vi "EXA SweepLoop.vi"(0 "Session In":refnum<visa-resource-name>="TCPIP0::169.254.70.120::inst0::INSTR", 1 "AVG":i32=4, 5 "Fstart":dbl=20.0 caption="RF_FREQ", 7 "Fstop":dbl=40.0 caption="RF_FREQ", 9 "Span(MHz)":dbl=1000.0, 11 "error in":errorcluster {"code" format="%.0x"}, 12 "RBW(Hz)":string="30") -> (3 "Max Freq/Ampl":dbl[](array[numeric]), 4 "VISA resource name out":refnum<visa-resource-name>, 15 "error out":errorcluster)   [LabVIEW 2018]
uses:
  Agilent MXA Series/Agilent MXA Series.lvlib
panel:
  out "RBW Read":dbl format="%#_6f"
  out "max value":dbl
  out "element":dbl=-103.604
  in  "stop":bool
  out "Mark Values":dbl[][](array[numeric])=[[20799.0, -104.6], [21873.0, -103.159], [22734.0, -104.034], [23667.0, -103.531], [25000.0, -101.288], [25000.0, -101.888], [26669.0, -103.797], [27125.0, -102.313], [28780.0, -103.097], [29360.0, -102.054], [30639.0, -102.503], [31191.0, -101.39], [32186.0, -101.846], [33650.0, -101.399], [34959.0, -100.372], [35490.0, -99.749], [36576.0, -98.986], [37771.0, -99.126], [38827.0, -99.917], [39888.0, -100.065]] format="%#.2f"
  out "RF_FREQ":dbl=27.5
  # "Sweep Segments and return the max value of concatenated seqments"
  # "Segemnts are = Span MHz Wide."
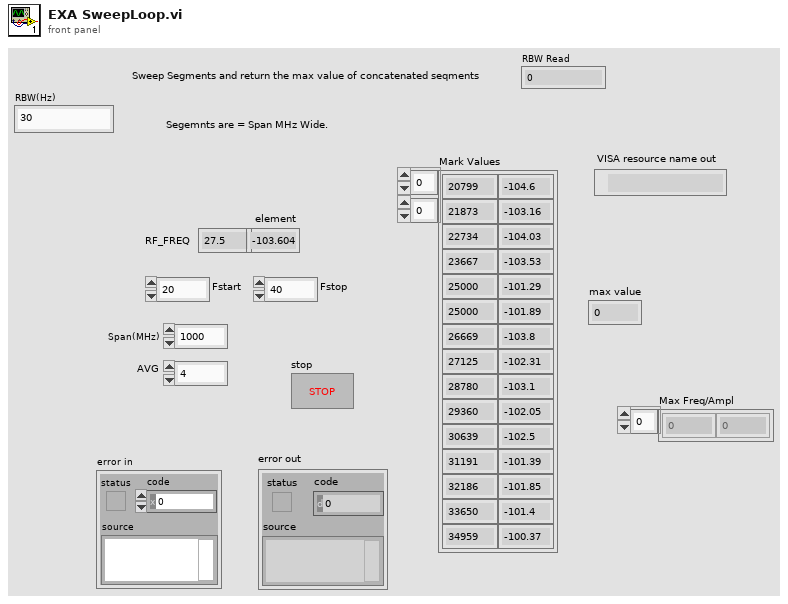
[diagram p1: front panel]
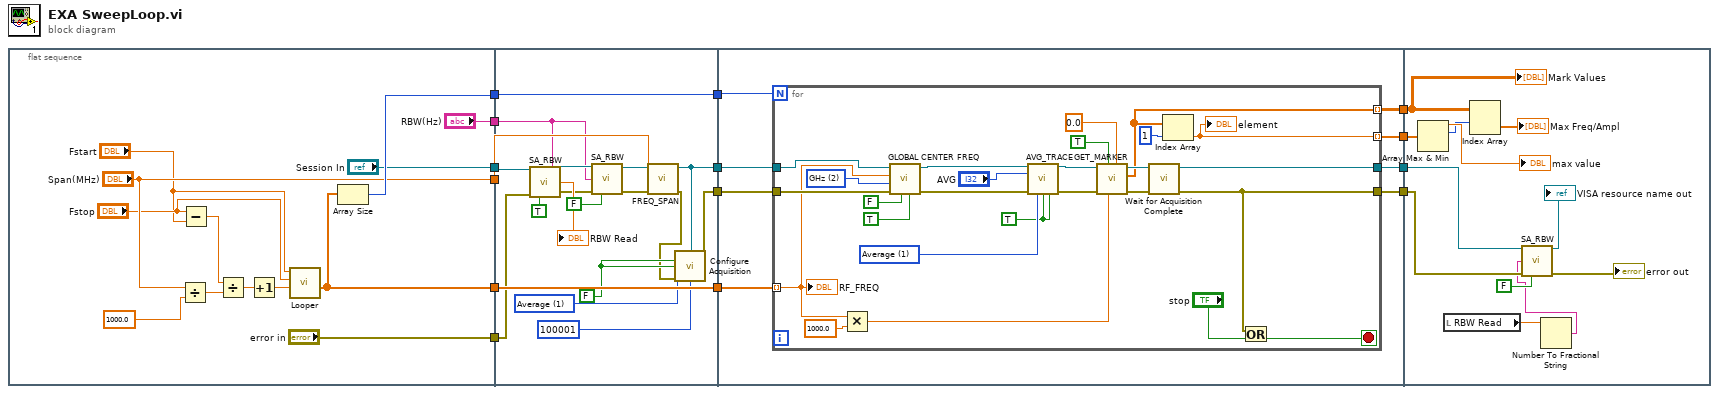
[diagram p0: block diagram]
diagram:
  n1 = flat-sequence {
    tunnel: [w22] -> w14
    tunnel: [w21] -> w13
    tunnel: ["Span(MHz)"] -> w12
    tunnel: ["Session In"] -> w11
    tunnel: ["error in"] -> w3
    tunnel: ["RBW(Hz)"] -> w1
    tunnel: w14 -> [w46]
    tunnel: w13 -> [w45]
    tunnel: w12 -> [w44]
    tunnel: w11 -> [w38]
    tunnel: [w46] -> w10
    tunnel: [w45] -> w9
    tunnel: [w28] -> w8
    tunnel: [w30] -> w7
    tunnel: w3 -> [w43]
    tunnel: w1 -> [w35]
    tunnel: w10 -> [w51]
    tunnel: w9 -> [w54]
    tunnel: w8 -> [w52]
    tunnel: w7 -> [w53]
    tunnel: [w50] -> w6
    tunnel: [w49] -> w5
    tunnel: [w48] -> w4
    tunnel: [w47] -> w2
    tunnel: w6 -> [w92]
    tunnel: w5 -> [w85]
    tunnel: w4 -> [w90]
    tunnel: w2 -> [w87]
    frame #0 {
      n2 = Divide(x="Span(MHz)", y=1000.0) -> (x/y=w23:dbl)
      n3 = Subtract(x="Fstop", y="Fstart") -> (x-y=w26:dbl)
      n4 = Divide(x=w26, y=w23) -> (x/y=w24:dbl)
      n5 = Increment(x=w24) -> (x+1=w25:dbl)
      n6 = call "Looper.vi"("Num Points"=w25, "Max"="Fstop", "Min"="Fstart") -> ("Result"=w22:dbl[])  [unwired: 7 in, 1 out]
      n7 = Array Size(array=w22) -> (size(s)=w21:i32)
    }
    frame #1 {
      w31 = FALSE ("Enable Continuous Sweep (T: Enable)")
      w32 = 1 items=["Normal", "Average", "Peak", "Sample", "Negative peak"] ("Manual Detector Type (0: Normal)")
      n8 = call "SA_RBW.vi"("Session In"=w38, "RBW(Hz)"=w35, "error in"=w43, "RO (T)"=TRUE) -> ("Session Out"=w39:refnum<visa-resource-name>, "RBW Read"=→"RBW Read":dbl, "error out"=w36:errorcluster)  [unwired: 7 in, 2 out]
      n9 = call "SA_RBW.vi"("Session In"=w39, "RBW(Hz)"=w35, "error in"=w36, "RO (T)"=FALSE) -> ("Session Out"=w40:refnum<visa-resource-name>, "error out"=w37:errorcluster)  [unwired: 7 in, 3 out]
      n10 = call "FREQ_SPAN.vi"("error in"=w37, "Span(MHz)"=w44, "Session In"=w40) -> ("error out"=w29:errorcluster, "Session Out"=w30:refnum<visa-resource-name>)  [unwired: 6 in, 1 out]
      n11 = call "Configure Acquisition.vi"("VISA resource name"=w30, "Enable Continuous Sweep (T: Enable)"=w31, "Auto Detector (T: Enable)"=w31, "Manual Detector Type (0: Normal)"=w32, "error in (no error)"=w29, "Sweep Points (1001)"=100001) -> ("error out"=w28:errorcluster)  [unwired: 8 in, 1 out]
    }
    frame #2 {
      n12 = for {
        N: w54 -> [_]
        tunnel: w53 -> [w80]
        tunnel: w52 -> [w79]
        tunnel: w51 -> [w61] mode=indexing
        tunnel: [w60] -> w50 mode=indexing
        tunnel: [w56] -> w49
        tunnel: [w58] -> w48 mode=indexing
        tunnel: [w55] -> w47
        stop <- w57 stop-if-true
        w74 = u16 2 items=["Hz", "MHz", "GHz"] ("Freq Units")
        w76 = TRUE ("AVG Restart (T)")
        w77 = 1 items=["Clear Write", "Average", "Maximum Hold", "Minimum Hold"] ("Trace Type (0: Clear Write)")
        n13 = Multiply(x=w61, y=1000.0) -> (x*y=w66:dbl)
        n14 = call "GLOBAL CENTER FREQ.vi"("Send OPC? (T)"=TRUE, "READ ONLY (T)"=FALSE ("bypass ESA Freq Set(t)"), "error in"=w79, "Freq Units"=w74, "SET CF ()"=w61, "Session In"=w80) -> ("error out"=w70:errorcluster, "Session Out"=w71:refnum<visa-resource-name>)  [unwired: 3 in, 1 out]
        n15 = call "AVG_TRACE.vi"("Session In"=w71, "AVG Count"="AVG", "error in"=w70, "Trace Type (0: Clear Write)"=w77, "AVG Restart (T)"=w76, "Send OPC? (T)"=w76) -> ("Session Out"=w72:refnum<visa-resource-name>, "error out"=w73:errorcluster)  [unwired: 8 in]
        n16 = call "GET_MARKER.vi"("offset"=0.0 ("out_cal_ampl"), "Set MKR Freq (MHz)"=w66, "Use PK Search (T)"=TRUE, "error in"=w73, "Session In"=w72) -> ("error out"=w64:errorcluster, "Mark Values"=w60:dbl[], "Session Out"=w63:refnum<visa-resource-name>)  [unwired: 3 in, 1 out]
        n17 = call "Wait for Acquisition Complete.vi"("error in (no error)"=w64, "VISA resource name"=w63) -> ("error out"=w56:errorcluster, "VISA resource name out"=w55:refnum<visa-resource-name>)  [unwired: 8 in]
        n18 = Index Array(array=w60, index=1) -> (element=w58:dbl)
        "element" <- w58
        n19 = Or(x=w56, y="stop") -> (x .or. y?=w57:bool)
        "RF_FREQ" <- w61
      }
    }
    frame #3 {
      n20 = Array Max & Min(array=w90) -> (max value=→"max value":dbl, max index (indices)=w88:i32)  [unwired: 2 out]
      n21 = local read "RBW Read"() -> (w82:dbl)
      n22 = Index Array(array=w92, index (row)=w88) -> (element=→"Max Freq/Ampl":dbl[])  [unwired: 1 in]
      n23 = Number To Fractional String(number=w82) -> (F-format string=w81:string)  [unwired: 3 in]
      n24 = call "SA_RBW.vi"("Session In"=w87, "RBW(Hz)"=w81, "error in"=w85, "RO (T)"=FALSE) -> ("Session Out"=→"VISA resource name out":refnum<visa-resource-name>, "error out"=→"error out":errorcluster)  [unwired: 7 in, 3 out]
      "Mark Values" <- w92
    }
  }
